vi "SetVisibleGraphCtrl.vi"(9 "on/off":bool, 10 "활성 플롯":u32, 11 "ref graph in":refnum<vi>) -> (3 "ref graph out":refnum<vi>)   [LabVIEW 2018, in "Library-Ctrl.lvlib"]
uses:
  Library-Ctrl.lvlib
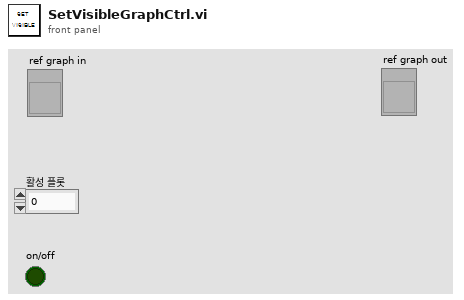
[diagram p1: front panel]
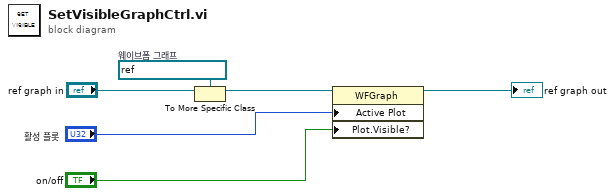
[diagram p0: block diagram]
diagram:
  w5 = refnum<vi> refnum  # 웨이브폼 그래프
  n1 = To More Specific Class(target class=w5, reference="ref graph in") -> (specific class reference=w4:refnum<vi>)  [unwired: 1 in, 1 out]
  n2 = property class="WFGraph"(reference=w4, "Active Plot"="활성 플롯", "Plot.Visible?"="on/off") -> (reference out=→"ref graph out":refnum<vi>)  [unwired: 1 in, 1 out]
